vi "BK Precision 913XX Timed Output.vi"() -> ()   [LabVIEW 2012]
doc: "This example shows how to configure the instrument's output to turn on for a specified amount of time using the output timer."
uses:
  <instrlib>/BK Precision 913XX/BK Precision 913XX.lvlib
panel:
  in  "Time (1s)":dbl=1.0 min=0.0 max=99999.9 step=1.0 format="%.1f"
  in  "Channel (1:1)":u16(ring)=1 items=["1"=1, "2"=2, "3"=3]
  in  "Current Limit (0.0 A)":dbl min=0.0 max=25.0 step=1.0 format="%.3f"
  in  "Voltage Level (0.0 V)":dbl format="%.3g"
  in  "VISA resource name":refnum<visa-resource-name>
  # "(c) 2015 B&K Precision Corporation.  ALL RIGHTS RESERVED."
  # "V"
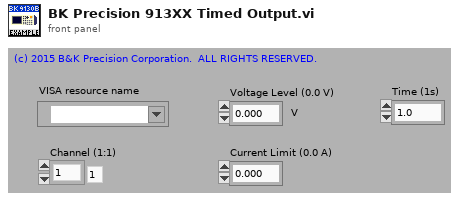
[diagram p1: front panel]
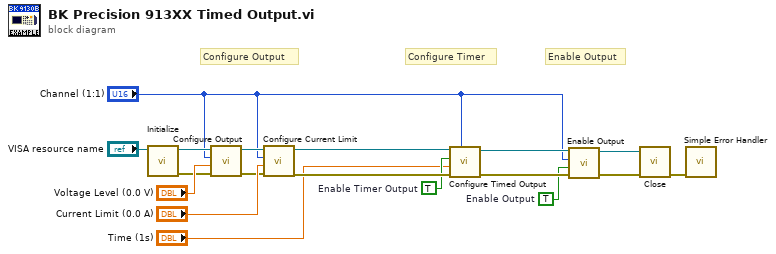
[diagram p0: block diagram]
diagram:
  w8 = TRUE  # Enable Timer Output
  w2 = TRUE  # Enable Output
  # "Enable Output"
  # "Configure Timer"
  # "Configure Output"
  n1 = call <instrlib>:"Initialize.vi"("VISA resource name"="VISA resource name") -> ("error out"=w11:errorcluster, "VISA resource name out"=w12:refnum<visa-resource-name>)  [unwired: 9 in]
  n2 = call <instrlib>:"Configure Output.vi"("error in (no error)"=w11, "Voltage Level (0.0 V)"="Voltage Level (0.0 V)", "Channel (1:1)"="Channel (1:1)", "VISA resource name"=w12) -> ("error out"=w13:errorcluster, "VISA resource name out"=w14:refnum<visa-resource-name>)  [unwired: 6 in]
  n3 = call <instrlib>:"Configure Current Limit.vi"("error in (no error)"=w13, "Current Limit (0.0 A)"="Current Limit (0.0 A)", "Channel (1:1)"="Channel (1:1)", "VISA resource name"=w14) -> ("error out"=w9:errorcluster, "VISA resource name out"=w10:refnum<visa-resource-name>)  [unwired: 6 in]
  n4 = call <instrlib>:"Configure Timed Output.vi"("Channel (1:1)"="Channel (1:1)", "error in (no error)"=w9, "Time (1s)"="Time (1s)", "Enable Timer Output (F: False)"=w8, "VISA resource name"=w10) -> ("error out"=w5:errorcluster, "VISA resource name out"=w6:refnum<visa-resource-name>)  [unwired: 5 in]
  n5 = call <instrlib>:"Enable Output.vi"("error in (no error)"=w5, "Enable Output (F: False)"=w2, "Channel (1:1)"="Channel (1:1)", "VISA resource name"=w6) -> ("error out"=w3:errorcluster, "VISA resource name out"=w4:refnum<visa-resource-name>)  [unwired: 6 in]
  n6 = call <instrlib>:"Close.vi"("error in (no error)"=w3, "VISA resource name"=w4) -> ("error out"=w17:errorcluster)  [unwired: 9 in]
  n7 = call <vilib>:"Simple Error Handler.vi"("error in (no error)"=w17) -> ()  [unwired: 4 in, 5 out]
